vi "Actor Core.vi"(8 "error in":errorcluster, 11 "DIMDemoClient in":refnum<class "DIMDemoClient.lvclass">) -> (0 "error out":errorcluster, 3 "Actor out":refnum<class "Actor.lvclass">)   [LabVIEW 2012, in "DimActorDemo.lvlib" / "DIMDemoClient.lvclass"]
doc: "(<B>Filename</B>: Actor Framework.lvlib:Actor.lvclass:Actor Core.vi)\n\nReceives messages to the actor, reacts to them, and initiates any error handling that may shut the actor down.\n\nDescendant classes may override this VI to append parallel tasks for the actor to complete while it handles messages. Overrides use the Call Parent Method node."
uses:
  DIMDemoClient.lvclass
  <vilib>/ActorFramework/Actor/Actor.lvclass
  SVN/LV2009/GPL/lib.lib/DimLVEvent/LVDimInterface/LVDimInterface.dim service type.ctl
  DIMActor/DIMActor/DIMActor.lvclass/DIMActor.ctl
  DIMDemoClient.lvclass/DIMDemoClient.ctl
  <vilib>/ActorFramework/Actor/Actor.lvclass/Actor.ctl
  <vilib>/ActorFramework/Message Enqueuer/Message Enqueuer.lvclass/Message Enqueuer.ctl
  DIMActor/DIMActor/DIMActor.lvclass
  <vilib>/ActorFramework/Message Enqueuer/Init from Existing Queue.vi
  <vilib>/ActorFramework/Message Enqueuer/Enqueue.vi
  <vilib>/ActorFramework/Message Priority Queue/Priority Enqueue.vi
  <vilib>/ActorFramework/Message Enqueuer/Message Enqueuer.lvclass
  <vilib>/ActorFramework/Stop Msg/Stop Msg.lvclass
  SVN/LV2009/GPL/lib.lib/DimLVEvent/LVDimInterface/LVDimInterface.lvlib
panel:
  out "Server Actor":string
  out "Name":string
  in  "Stop Button":bool
  in  "Send Command":bool
  out "DemoService":i32=-2
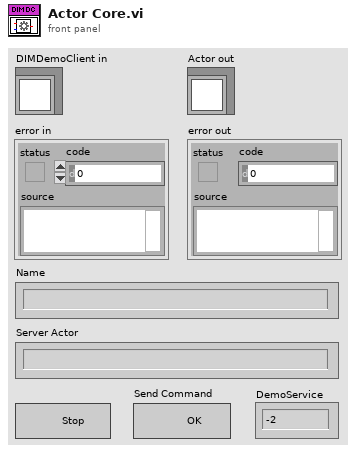
[diagram p1: front panel]
types:
  T1 = typedef "LVDimInterface.lvlib/LVDimInterface.dim service type.ctl" = u16
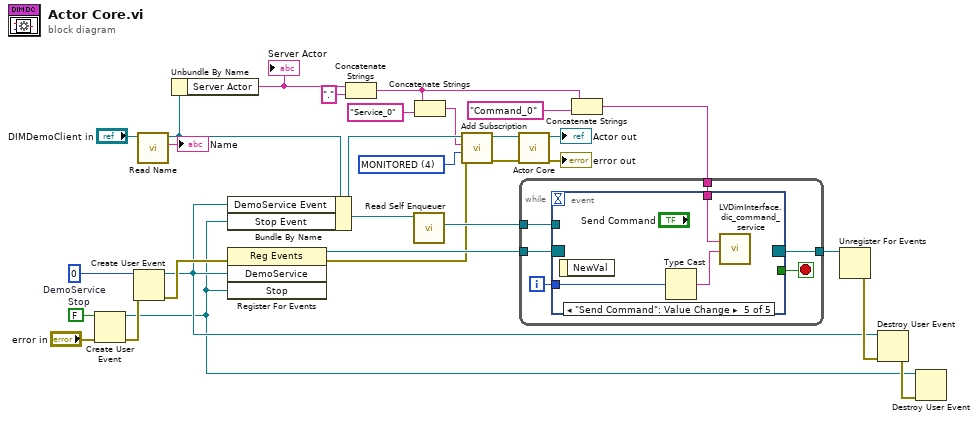
[diagram p0: block diagram]
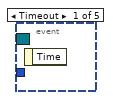
[diagram p2: hidden frame]
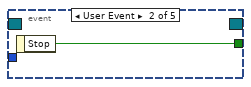
[diagram p3: hidden frame]
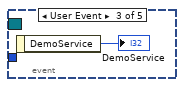
[diagram p4: hidden frame]
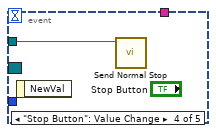
[diagram p5: hidden frame]
diagram:
  w24 = FALSE  # Stop
  w25 = 0  # DemoService
  w26 = T1 4 items=["ONCE_ONLY"=1, "TIMED"=2, "MONITORED"=4] ("Service Type")
  n1 = Create User Event(user event datatype=w24, error in="error in") -> (user event=w11:refnum<user-event>, error out=w23:errorcluster)
  n2 = Create User Event(user event datatype=w25, error in=w23) -> (user event=w12:refnum<user-event>, error out=w22:errorcluster)
  n3 = call "Read Name.vi"("DIMActor in"="DIMDemoClient in") -> ("Name"=→"Name":string, "DIMActor out"=w2:refnum<class "DIMDemoClient.lvclass">)  [unwired: 8 in, 1 out]
  n4 = Unbundle By Name(w2) -> ("Server Actor"=w4:string)
  "Server Actor" <- w4
  n5 = Bundle By Name(cluster=w2, "DemoService Event"=w12, "Stop Event"=w11) -> (w13:refnum<class "DIMDemoClient.lvclass">)
  n6 = register-events(error in=w22, w12, w11) -> (reference out=w21:refnum<event-registration>, error out=w15:errorcluster)  [unwired: 1 in]
  n7 = Concatenate Strings(w4, "." ("string")) -> (w6:string)
  n8 = call <vilib>:"Read Self Enqueuer.vi"("Actor"=w13) -> ("Self Enqueuer"=w20:refnum<class "Message Enqueuer.lvclass">)  [unwired: 10 in]
  n9 = Concatenate Strings(w6, "Service_0" ("Subscription Name")) -> (w8:string)
  n10 = call "Add Subscription.vi"("error in (no error)"=w15, "Service Type"=w26, "Subscription Name"=w8, "DIMActor in"=w13) -> ("error out"=w14:errorcluster, "DIMActor out"=w27:refnum<class "DIMDemoClient.lvclass">)  [unwired: 6 in]
  n11 = call-parent "Actor Core.vi"("error in"=w14, "DIMActor in"=w27) -> ("error out"=→"error out":errorcluster, "Actor out"=→"Actor out":refnum<class "Actor.lvclass">)  [unwired: 8 in]
  n12 = Concatenate Strings(w6, "Command_0" ("Command Name")) -> (w5:string)
  n13 = while {
    tunnel: w21 -> [w35]
    tunnel: w20 -> [w33]
    tunnel: [w32] -> w19
    tunnel: w5 -> [w30]
    i -> [w31]
    stop <- w34 stop-if-true
    n14 = event shown="[4] \"Send Command\": Value Change" {
      selector: w35 -> [_ _ _ _ _]
      dyn-events: [_ _ _ _ _] -> w32
      timeout: _ -> [_ _ _ _ _]
      tunnel: [_ w36 _ _ _] -> w34
      tunnel: w33 -> [_ _ _ w38 _]
      tunnel: w31 -> [_ _ _ _ w41]
      tunnel: w30 -> [_ _ _ _ w39]
      event Timeout {
        n15 = event-data() -> ()  [unwired: 1 in, 1 out]
      }
      event User Event {
        n16 = event-data() -> ("Stop"=w36:bool)  [unwired: 1 in]
      }
      event User Event {
        n17 = event-data() -> ("DemoService"=→"DemoService":i32)  [unwired: 1 in]
      }
      event "Stop Button": Value Change {
        n18 = event-data() -> ()  [unwired: 1 in, 1 out]
        n19 = call <vilib>:"Send Normal Stop.vi"("Message Enqueuer"=w38) -> ()  [unwired: 10 in, 1 out]
      }
      event "Send Command": Value Change {
        n20 = event-data() -> ()  [unwired: 1 in, 1 out]
        n21 = Type Cast(x=w41) -> (*(type *) &x=w40:string)  [unwired: 1 in]
        n22 = call "LVDimInterface.dic_command_service.vi"("commandName"=w39, "data"=w40) -> ()  [unwired: 16 in, 2 out]
      }
    }
  }
  n23 = Unregister For Events(event registration refnum=w19) -> (error out=w18:errorcluster)  [unwired: 1 in]
  n24 = Destroy User Event(user event=w12, error in=w18) -> (error out=w17:errorcluster)
  n25 = Destroy User Event(user event=w11, error in=w17) -> ()  [unwired: 1 out]
